vi "WVDIAL_GlobalVariables.vi"() -> ()   [LabVIEW 2012]
uses:
  TypeDefinitions.llb/TypeDef_MainControlSystem.ctl
panel:
  in  "Tab Control":enum32{"Main Globals", "Laser Globals"}(tab)
  in  "ChildTimeout (sec)":dbl=5.0
  out "ChildAbort":bool
  in  "VI Timeout (min)":dbl=5.0
  in  "Global File Paths":path[](array[path])=[path "/Freundlein/Users/Bobby/Desktop/NCARLabviewTesting/Log.llb/Log_SetUserComment.vi", path "/Freundlein/Users/Bobby/Desktop/NCARLabviewTesting/Idle.llb/Idle_Password.vi"]
  out "RunAsChild":bool
  out "GlobalStop":bool
  in  "PermissionLevel":i32
  out "Children Details":T2(array[cluster])
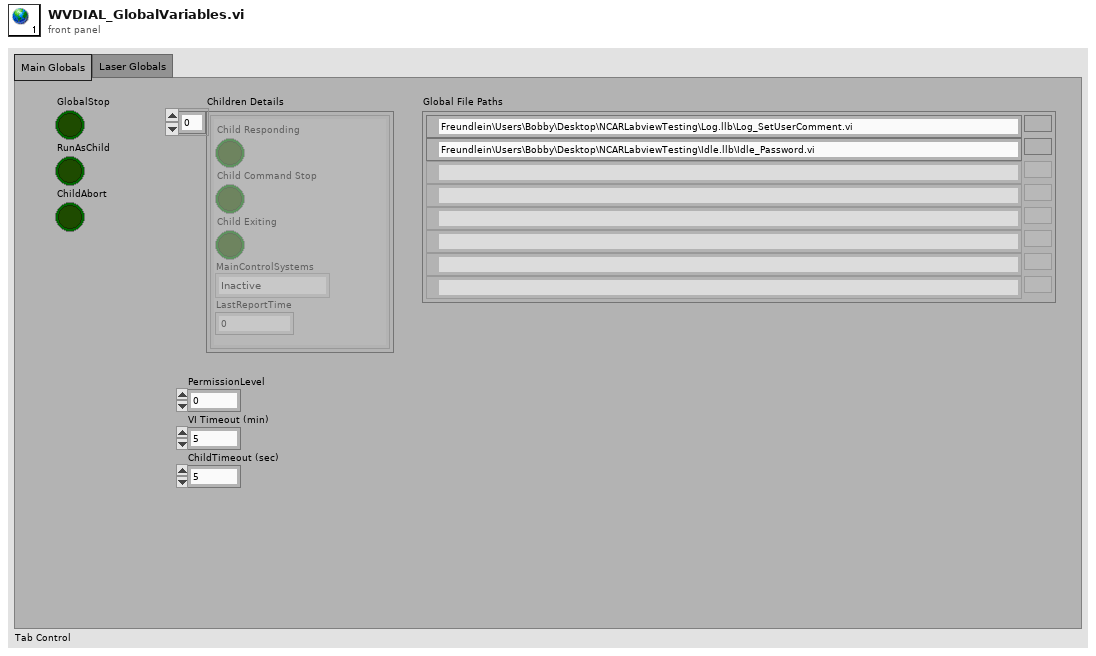
[diagram p1: front panel]
types:
  T1 = typedef "TypeDef_MainControlSystem.ctl" = enum16{"Inactive", "MCSControl", "MCSDisplay", "LaserControl", "LaserLocking", "WeatherStation", "DataDisplay", "Template"}
  T2 = cluster{"Child Command Stop":bool, "Child Responding":bool, "MainControlSystems":T1, "LastReportTime":dbl, "Child Exiting":bool}[]
diagram:
